vi "Error Terminal on Con Pane.vi"(8 "error in":errorcluster, 11 "VI in":refnum<vi>) -> (0 "error out":errorcluster, 3 "Error Terminal on Con Pane?":bool)   [LabVIEW 2024]
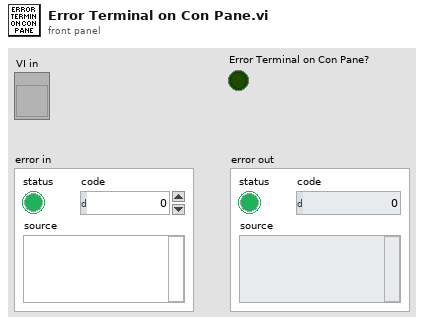
[diagram p1: front panel]
types:
  T1 = enum32{"invalid VI type", "Standard VI", "Control VI", "Global VI", "Polymorphic VI", "Configuration VI", "SubSystem", "Facade VI", "Method VI", "Statechart Diagram VI"}
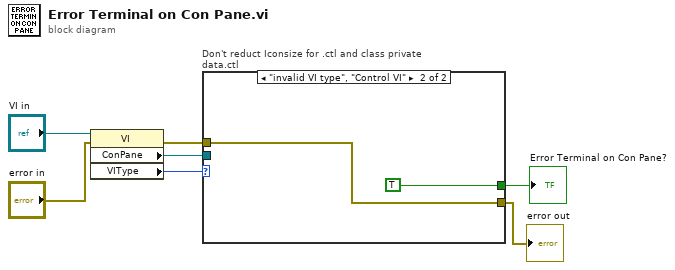
[diagram p0: block diagram]
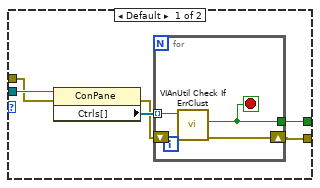
[diagram p2: hidden frame]
diagram:
  n1 = property class="VI"(reference="VI in", error in="error in") -> (error out=w4:errorcluster, "ConPane"=w7:refnum<vi>, "VIType"=w5:T1)  [unwired: 1 out]
  n2 = case "Don't reduct Iconsize for .ctl and class private data.ctl" shown="\"invalid VI type\", \"Control VI\"" w5 {
    tunnel: w7 -> [w13 _]
    tunnel: [w9 TRUE] -> w3
    tunnel: w4 -> [w11 w18]
    tunnel: [w8 w18] -> w2
    frame Default {
      n3 = property class="ConPane"(reference=w13, error in=w11) -> (error out=w10:errorcluster, "Ctrls[]"=w12:refnum<vi>[])  [unwired: 1 out]
      n4 = for {
        tunnel: w12 -> [w17] mode=indexing
        shift-right: [w16] -> w8
        shift-left: w10 -> [w15]
        tunnel: [w14] -> w9
        stop <- w14 stop-if-true
        n5 = call <vilib>:"VIAnUtil Check If ErrClust.vi"("error in (no error)"=w15, "Control in"=w17) -> ("error out"=w16:errorcluster, "Is error cluster?"=w14:bool)  [unwired: 7 in, 1 out]
      }
    }
    frame "invalid VI type", "Control VI" {
    }
  }
  "Error Terminal on Con Pane?" <- w3
  "error out" <- w2
